vi "Readjust Voltage.vi"(8 "error in (no error)":errorcluster, 10 "New Voltage":dbl, 11 "object in":refnum<class "Pulsetrain Config.lvclass">) -> (0 "error out":errorcluster, 3 "object out":refnum<class "Pulsetrain Config.lvclass">)   [LabVIEW 2023, in "Teledyne-T3AFG120.lvlib" / "Pulsetrain Config.lvclass"]
uses:
  Pulsetrain Config.lvclass
  Pulsetrain Config.lvclass/Pulsetrain Config.ctl
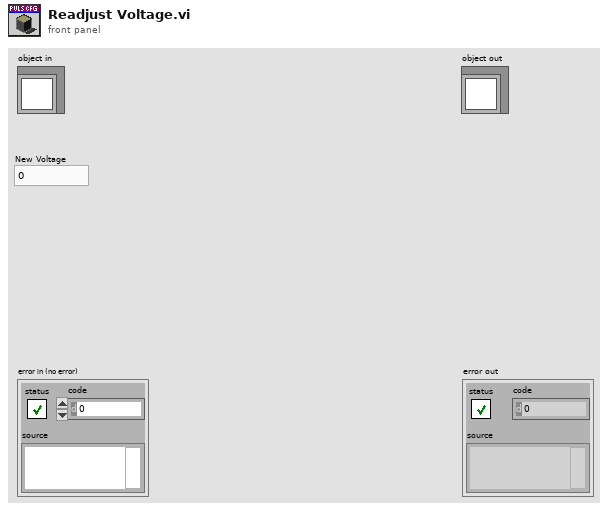
[diagram p1: front panel]
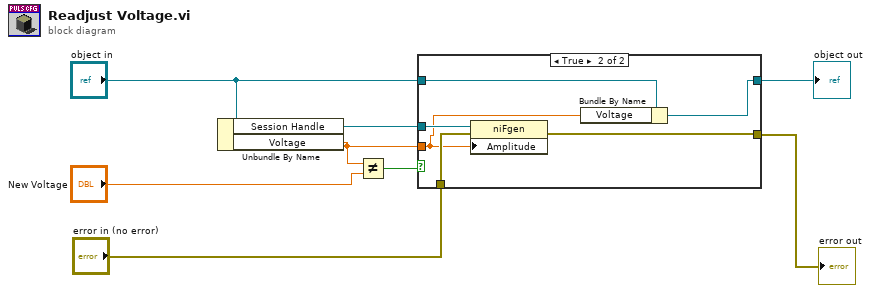
[diagram p0: block diagram]
diagram:
  n1 = Unbundle By Name("object in") -> ("Session Handle"=w6:refnum<k15>, "Voltage"=w4:dbl)
  n2 = Not Equal?(x=w4, y="New Voltage") -> (x != y?=w5:bool)
  n3 = case shown="True" w5 {
    tunnel: "error in (no error)" -> [w10 w16]
    tunnel: w6 -> [_ w15]
    tunnel: w4 -> [_ w12]
    tunnel: [w10 w14] -> w3
    tunnel: "object in" -> [w9 w13]
    tunnel: [w9 w11] -> w1
    frame False {
    }
    frame True {
      n4 = property class="niFgen"(reference=w15, error in=w16, "Amplitude"=w12) -> (error out=w14:errorcluster)  [unwired: 1 out]
      n5 = Bundle By Name(cluster=w13, "Voltage"=w12) -> (w11:refnum<class "Pulsetrain Config.lvclass">)
    }
  }
  "error out" <- w3
  "object out" <- w1
